vi "ILD1420_Global.vi"() -> ()   [LabVIEW 2018]
panel:
  out "First run":bool=TRUE
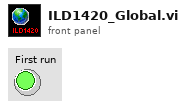
[diagram p1: front panel]
diagram:
